vi "Merge VeriStand .NET Error.vi"(8 "error in":errorcluster, 11 "error":refnum<k39>) -> (0 "error out":errorcluster)   [LabVIEW 2027, in "Embedded Data Logger Scripting.lvlib"]
uses:
  Embedded Data Logger Scripting.lvlib
  C:/NetCore/niveristand-embedded-data-logger-custom-device/Source/Scripting/Utility/Merge VeriStand .NET Error.vi/NationalInstruments.VeriStand
  NationalInstruments.VeriStand
  C:/NetCoreDLL/NationalInstruments.VeriStand.dll
  NetCoreDLL/NationalInstruments.VeriStand.dll
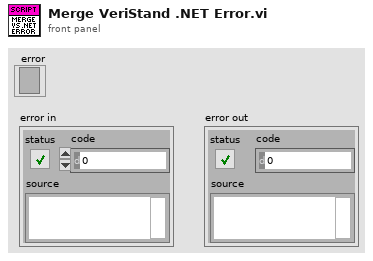
[diagram p1: front panel]
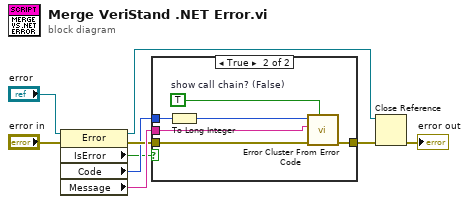
[diagram p0: block diagram]
diagram:
  n1 = property class="Error"(reference="error", error in="error in") -> (reference out=w7:refnum<k39>, error out=w8:errorcluster, "IsError"=w1:bool, "Code"=w2:u32, "Message"=w9:string)
  n2 = case shown="True" w1 {
    tunnel: w9 -> [_ w15]
    tunnel: w8 -> [w10 w14]
    tunnel: [w10 w13] -> w5
    tunnel: w2 -> [_ w12]
    frame False {
    }
    frame True {
      w11 = TRUE  # show call chain? (False)
      n3 = To Long Integer(number=w12) -> (32bit integer=w16:i32)
      n4 = call <vilib>:"Error Cluster From Error Code.vi"("show call chain? (False)"=w11, "error in (no error)"=w14, "error message (\"\")"=w15, "error code (0)"=w16) -> ("error out"=w13:errorcluster)  [unwired: 5 in]
    }
  }
  n5 = Close Reference(reference=w7, error in (no error)=w5) -> (error out=→"error out":errorcluster)
